vi "Timestamp to EPICS Timestamp.vi"(0 "timestamp":timestamp, 1 "user tag":i32) -> (2 "epics timestamp":T1)   [LabVIEW 2020, in "PV Access.lvlib" / "PV Data.lvlib"]
uses:
  PV Data.lvlib
  EPICS Timestamp.ctl
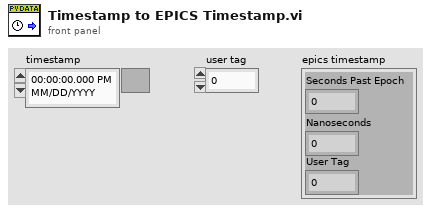
[diagram p1: front panel]
types:
  T1 = typedef "PV Access.lvlib/PV Data.lvlib/EPICS Timestamp.ctl" = cluster{"Seconds Past Epoch":i64, "Nanoseconds":i32, "User Tag":i32}
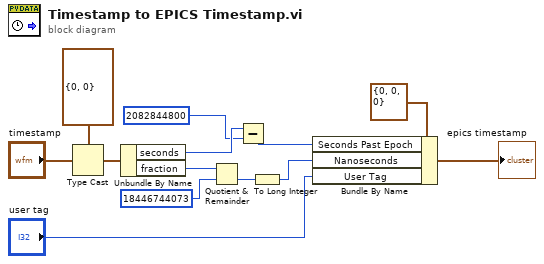
[diagram p0: block diagram]
diagram:
  n1 = Type Cast(type=cluster{"seconds":i64, "fraction":u64} {"seconds"=0, "fraction"=0}, x="timestamp") -> (*(type *) &x=w11:cluster{"seconds":i64, "fraction":u64})
  n2 = Unbundle By Name(w11) -> ("seconds"=w10:i64, "fraction"=w5:u64)
  n3 = Quotient & Remainder(x=w5, y=u64 18446744073) -> (floor(x/y)=w3:u64)  [unwired: 1 out]
  n4 = Subtract(x=w10, y=i64 2082844800) -> (x-y=w7:i64)
  n5 = To Long Integer(number=w3) -> (32bit integer=w2:i32)
  n6 = Bundle By Name(cluster=T1 {"Seconds Past Epoch"=0, "Nanoseconds"=0, "User Tag"=0} ("timestamp"), "Seconds Past Epoch"=w7, "Nanoseconds"=w2, "User Tag"="user tag") -> (→"epics timestamp":T1)
